vi "Launch LabActor.vi"() -> ()   [LabVIEW 2016]
uses:
  LabActor/LabActor.lvclass
  C:/github/LabActor/Controllers/Application Controller/Application Controller.lvclass
  Controllers/Application Controller/Load App.vi
  Controllers/Application Controller/Application Controller.lvclass
panel:
  out "Path":string
  out "Waiting Lights":T1
  out "Current action:":string
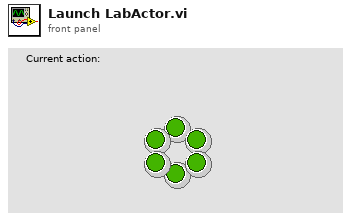
[diagram p1: front panel]
types:
  T1 = cluster{"DNL_wait 1":bool, "DNL_wait 1":bool, "DNL_wait 1":bool, "DNL_wait 1":bool, "DNL_wait 1":bool, "DNL_wait 1":bool}
  T2 = cluster{"[0]":bool, "[1]":bool, "[2]":bool, "[3]":bool, "[4]":bool, "[5]":bool}
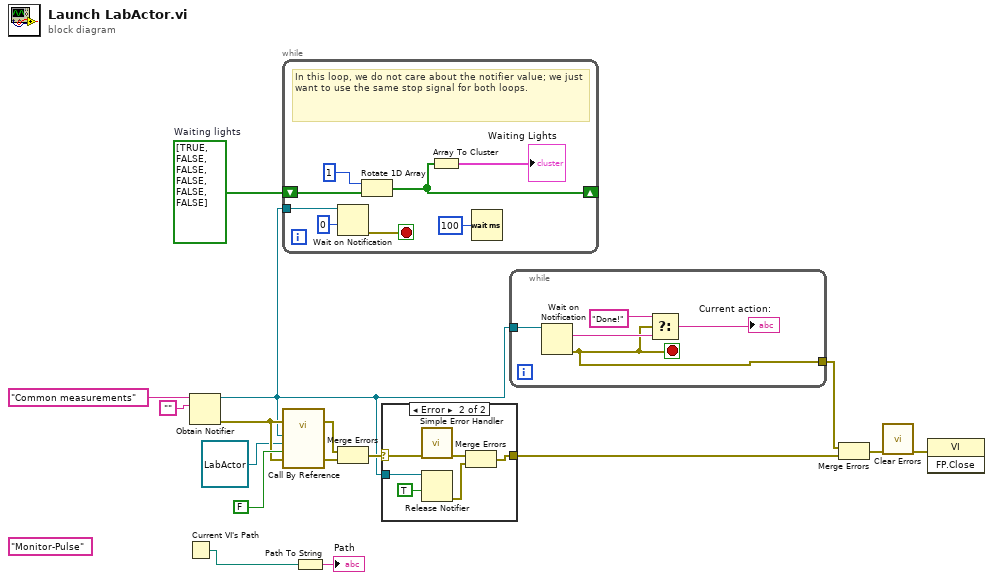
[diagram p0: block diagram]
diagram:
  (unwired) "Monitor-Pulse" ("Name")
  w5 = bool[] [TRUE, FALSE, FALSE, FALSE, FALSE, FALSE]  # Waiting lights
  n1 = Current VI's Path() -> (path=w2:path)
  n2 = Obtain Notifier(name (unnamed)="Common measurements", notification data type="") -> (notifier out=w3:refnum<notifier>, error out=w11:errorcluster)  [unwired: 2 in, 1 out]
  n3 = while {
    shift-right: [w18] -> _
    shift-left: w5 -> [w20]
    tunnel: w3 -> [w22]
    stop <- w24 stop-if-true
    # "In this loop, we do not care about the notifier value; we just want to use the same stop signal for both loops."
    n4 = Wait on Notification(notifier=w22, timeout in ms (-1)=0) -> (error out=w24:errorcluster)  [unwired: 2 in, 3 out]
    n5 = Rotate 1D Array(1:w20, 2:1 ("n")) -> (0:w18:bool[])
    n6 = Array To Cluster(array=w18) -> (cluster=→"Waiting Lights":T2)
    n7 = Wait (ms)(milliseconds to wait=u32 100) -> ()  [unwired: 1 out]
  }
  n8 = call-by-ref "?"(error in=w11, "Error In"=w11, "Open Actor Core front panel? (F)"=FALSE, "Application Controller.lvclass"=refnum<class "LabActor.lvclass"> refnum ("LabActor.lvclass"), "Status Notifier"=w3) -> (error out=w14:errorcluster, "Error Out"=w10:errorcluster)  [unwired: 8 in, 1 out]
  n9 = Path To String(path=w2) -> (string=→"Path":string)
  n10 = Merge Errors(w14, w10) -> (w15:errorcluster)
  n11 = case shown="Error" w15 {
    selector: w15 -> [w25 w31]
    tunnel: [w25 w28] -> w8
    tunnel: w3 -> [_ w30]
    frame No Error {
    }
    frame Error {
      n12 = call <vilib>:"Simple Error Handler.vi"("error in (no error)"=w31) -> ("error out"=w29:errorcluster)  [unwired: 4 in, 4 out]
      n13 = Release Notifier(notifier=w30, force destroy? (F)=TRUE) -> (error out=w27:errorcluster)  [unwired: 1 in, 2 out]
      n14 = Merge Errors(w29, w27) -> (w28:errorcluster)
    }
  }
  n15 = while {
    tunnel: w3 -> [w36]
    tunnel: [w32] -> w6
    stop <- w32 stop-if-true
    n16 = Wait on Notification(notifier=w36) -> (notification=w34:string, error out=w32:errorcluster)  [unwired: 3 in, 2 out]
    n17 = Select(t="Done!" ("notification"), s=w32, f=w34) -> (s? t:f=→"Current action:":string)
  }
  n18 = Merge Errors(w6, w8) -> (w7:errorcluster)
  n19 = call <vilib>:"Clear Errors.vi"("error in (no error)"=w7) -> ("error out"=w16:errorcluster)  [unwired: 5 in, 1 out]
  n20 = invoke class="VI" method="FP.Close"(error in=w16) -> ()  [unwired: 2 in, 3 out]
